vi "Persist New Entity.vi"(8 "error in (no error)":errorcluster, 10 "New Entity":refnum<class "Entity.lvclass">, 11 "Entity Manager in":refnum<class "Entity Manager.lvclass">) -> (0 "error out":errorcluster, 2 "Entity":refnum<class "Entity.lvclass">, 3 "Entity Manager out":refnum<class "Entity Manager.lvclass">)   [LabVIEW 2022 SP3, in "Conditum.lvlib" / "Entity Manager.lvclass"]
uses:
  Entity Manager.lvclass
  Entity/Entity.lvclass
  Entity/Entity.lvclass/Entity.ctl
  Columns/ID/ID.lvclass/ID.ctl
  Columns/ID/Set.vi
  Entity Manager.lvclass/Entity Manager.ctl
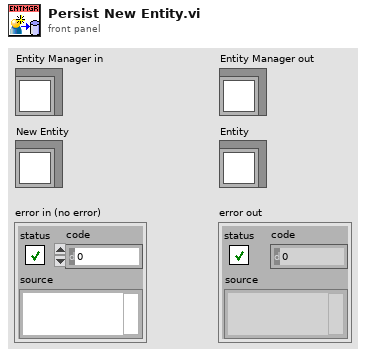
[diagram p1: front panel]
types:
  T1 = typedef "Conditum.lvlib/Entity ID.ctl" = i64
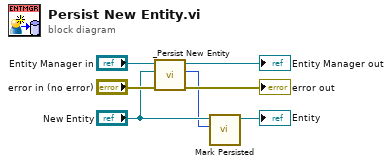
[diagram p0: block diagram]
diagram:
  n1 = call "_Persist New Entity.vi"("error in (no error)"="error in (no error)", "New Entity"="New Entity", "Entity Manager in"="Entity Manager in") -> ("error out"=→"error out":errorcluster, "Entity ID"=w2:T1, "Entity Manager out"=→"Entity Manager out":refnum<class "Entity Manager.lvclass">)  [unwired: 6 in]
  n2 = call "Mark Persisted.vi"("Entity ID"=w2, "Entity in"="New Entity") -> ("Entity out"=→"Entity":refnum<class "Entity.lvclass">)  [unwired: 9 in]
